vi "Delete.vi"(6 "commandTimeout":i32, 8 "error in (no error)":errorcluster, 9 "DynamicParameters":refnum<class "DynamicParameters.lvclass">, 10 "TableName":string, 11 "SqlMapper in":refnum<class "SqlMapper.lvclass">) -> (0 "error out":errorcluster, 1 "AffectedRows":i32, 3 "SqlMapper out":refnum<class "SqlMapper.lvclass">)   [LabVIEW 2020, in "ORM.lvlib" / "SqlMapper.lvclass"]
uses:
  SqlMapper.lvclass
  DynamicParameters/DynamicParameters.lvclass
  SqlMapper.lvclass/SqlMapper.ctl
  DbConnection/DbConnection.lvclass
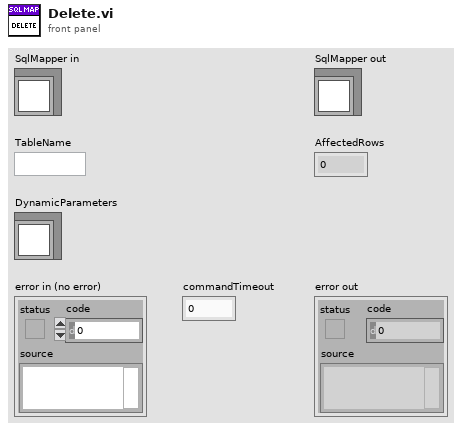
[diagram p1: front panel]
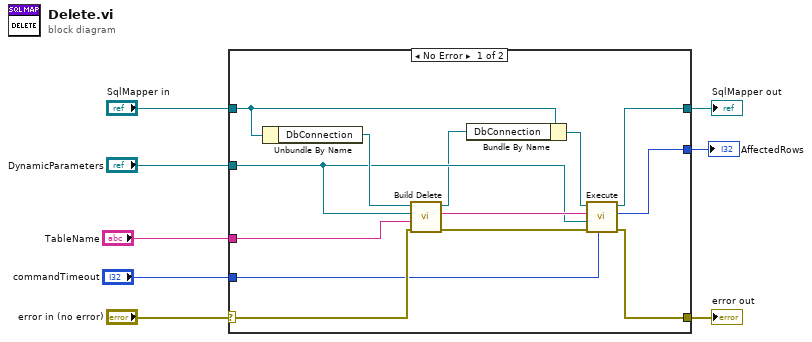
[diagram p0: block diagram]
diagram:
  n1 = case shown="No Error" "error in (no error)" {
    selector: "error in (no error)" -> [w16 w23]
    tunnel: [w11 w23] -> w7
    tunnel: [w13 w22] -> w5
    tunnel: "SqlMapper in" -> [w19 w22]
    tunnel: "DynamicParameters" -> [w17 _]
    tunnel: "TableName" -> [w20 _]
    tunnel: "commandTimeout" -> [w14 _]
    tunnel: [w12 _] -> w1
    frame No Error {
      n2 = Unbundle By Name(w19) -> ("DbConnection"=w21:refnum<class "DbConnection.lvclass">)
      n3 = call-dynamic "Build Delete.vi"("error in (no error)"=w16, "tableName"=w20, "DynamicParameters in"=w17, "DbConnection in"=w21) -> ("error out"=w15:errorcluster, "Query"=w18:string, "DbConnection out"=w9:refnum<class "DbConnection.lvclass">)  [unwired: 5 in]
      n4 = Bundle By Name(cluster=w19, "DbConnection"=w9) -> (w10:refnum<class "SqlMapper.lvclass">)
      n5 = call-dynamic "Execute.vi"("commandTimeout"=w14, "error in (no error)"=w15, "DynamicParameters"=w17, "sql"=w18, "SqlMapper in"=w10) -> ("error out"=w11:errorcluster, "affectedRows"=w12:i32, "SqlMapper out"=w13:refnum<class "SqlMapper.lvclass">)  [unwired: 4 in]
    }
    frame Error {
    }
  }
  "error out" <- w7
  "SqlMapper out" <- w5
  "AffectedRows" <- w1
